vi "HEWH Date Sort.vi"(8 "error in (no error)":errorcluster, 10 "FHR Test Date":string, 11 "24 Hour Test Date":string) -> (0 "error out":errorcluster, 3 "Earliest Date":string)   [LabVIEW 2023]
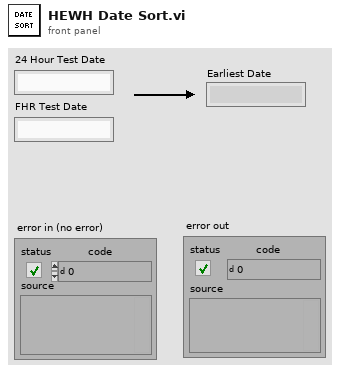
[diagram p1: front panel]
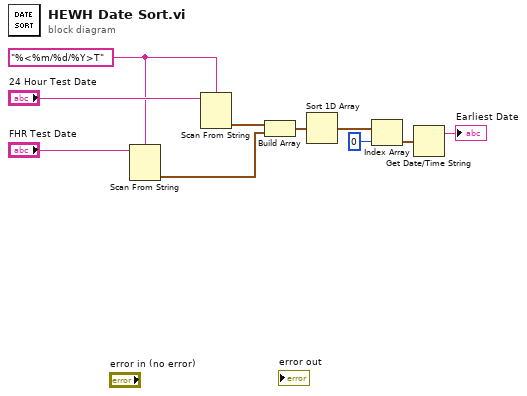
[diagram p0: block diagram]
diagram:
  w8 = "%<%m/%d/%Y>T" ("format string")
  n1 = Scan From String(format string=w8, input string="FHR Test Date") -> (output 1=w6:timestamp)  [unwired: 3 in, 3 out]
  n2 = Scan From String(format string=w8, input string="24 Hour Test Date") -> (output 1=w7:timestamp)  [unwired: 3 in, 3 out]
  n3 = Build Array(w7, w6) -> (w5:timestamp[])
  n4 = Sort 1D Array(array=w5) -> (sorted array=w4:timestamp[])
  n5 = Index Array(array=w4, index=0) -> (element=w2:timestamp)
  n6 = Get Date/Time String(seconds (now)=w2) -> (date string=→"Earliest Date":string)  [unwired: 2 in, 1 out]
